vi "sub_waypoint_load.vi"(11 "path":path) -> (3 "XY 그래프":cluster{"X":dbl, "Y":dbl}[](graph))   [LabVIEW 2019]
panel:
  out "read":string
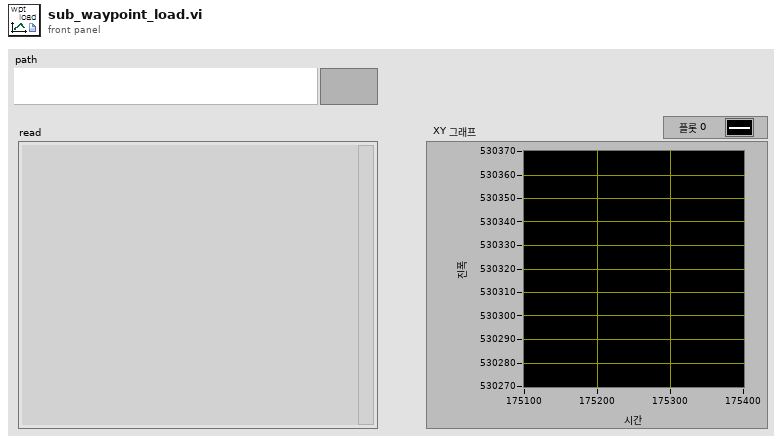
[diagram p1: front panel]
types:
  T1 = cluster{"배열 타입(2D Dbl)[0]":dbl, "배열 타입(2D Dbl)[1]":dbl}[]
  T2 = cluster{"배열 타입(2D Dbl)[0]":dbl, "배열 타입(2D Dbl)[1]":dbl}
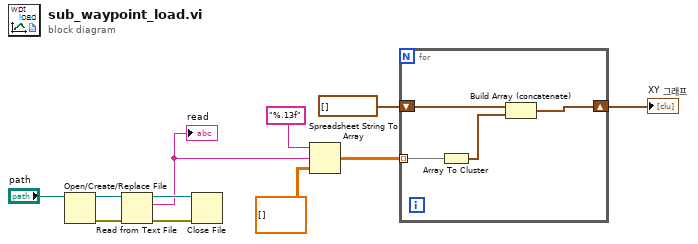
[diagram p0: block diagram]
diagram:
  n1 = Open/Create/Replace File(file path (use dialog)="path") -> (refnum out=w8:refnum<file>, error out=w11:errorcluster)  [unwired: 5 in, 1 out]
  n2 = Read from Text File(file (use dialog)=w8, error in=w11) -> (refnum out=w9:refnum<file>, text=w7:string, error out=w10:errorcluster)  [unwired: 2 in, 1 out]
  "read" <- w7
  n3 = Close File(refnum=w9, error in=w10) -> ()  [unwired: 2 out]
  n4 = Spreadsheet String To Array(format string="%.13f" ("포맷 문자열"), spreadsheet string=w7, array type (2D Dbl)=dbl[][] [] ("배열 타입(2D Dbl)")) -> (array=w4:dbl[][])  [unwired: 1 in]
  n5 = for {
    tunnel: w4 -> [w15] mode=indexing
    shift-right: [w13] -> w2
    shift-left: T1 [] -> [w12]
    n6 = Array To Cluster(array=w15) -> (cluster=w14:T2)
    n7 = Build Array (concatenate)(w12, w14) -> (w13:T1)
  }
  "XY 그래프" <- w2
